vi "Global constant.vi"() -> ()   [LabVIEW 2013]
panel:
  in  "Name":string
  out "Info":cluster{"PASS":u32, "Total":u32, "Rate":dbl}
  in  "Lock":string(combo)="port0/line0"
  in  "DAQ":tag="Dev7"
  in  "Test Time":string
  in  "CAN_Channel":i32
  in  "CAN_Device":i32
  out "Backup_path":path
  out "Mis_path":path
  in  "BIO2":i32
  in  "BIO1":i32
  out "FailGoOn":bool
  out "MAC ID":string
  in  "DMM":refnum<visa-resource-name>="COM12"
  in  "Spare":refnum<visa-resource-name>="COM12"
  in  "DC Souse":refnum<visa-resource-name>="COM12"
  in  "ZY_Relay":refnum<visa-resource-name>="COM12"
  out "SN":string
  out "Result":bool
  in  "Model":string
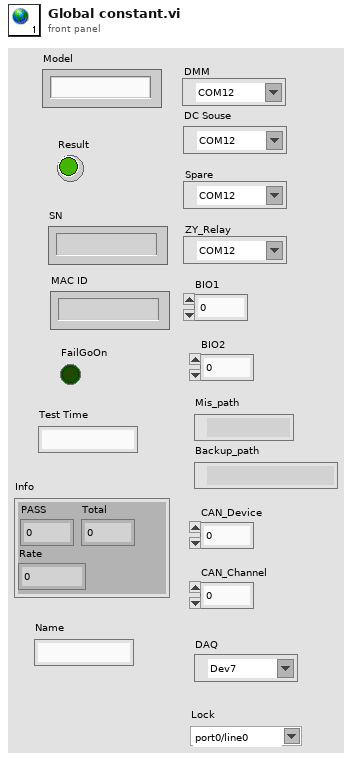
[diagram p1: front panel]
diagram:
